vi "activeXtest2015.vi"() -> ()   [LabVIEW 2015]
uses:
  <vilib>/Utility/NIReport.llb/NI_report.lvclass
  <vilib>/addons/_office/NI_ReportGenerationToolkit.lvlib
  <vilib>/Utility/NIReport.llb/Excel/NI_Excel.lvclass
panel:
  out "cell's name":string
  in  "Select Worksheet":i32
  in  "start (-1, -1) 2":cluster{"row":i32, "column":i32}={"row"=-1, "column"=-1}
  out "Worksheet Name":string
  out "Worksheet Names":string[](array[string])
  out "worksheets count":i32
  in  "end (-1, -1)":cluster{"row":i32, "column":i32}={"row"=-1, "column"=-1}
  in  "start (-1, -1)":cluster{"row":i32, "column":i32}={"row"=15, "column"=13}
  in  "report file path":path=path "D:/Cascade/templates/Groundwater Profiling Log_empty_1.xlsx"
  out "error out":errorcluster
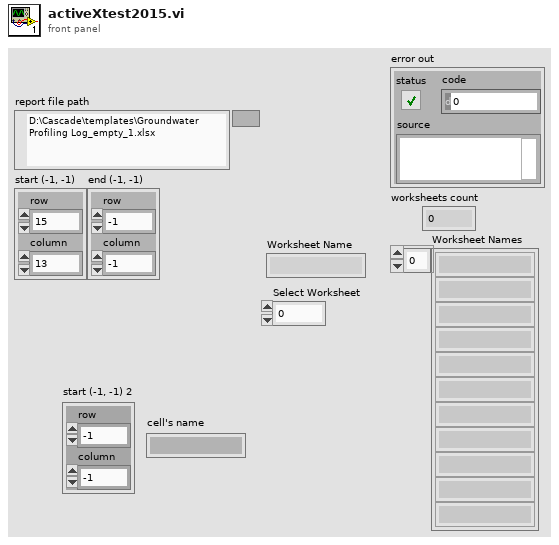
[diagram p1: front panel]
types:
  T1 = enum16{"Standard Report", "HTML", "Word", "Excel"}
  T2 = cluster{"on/off":bool, "weight":i32, "color":u32}
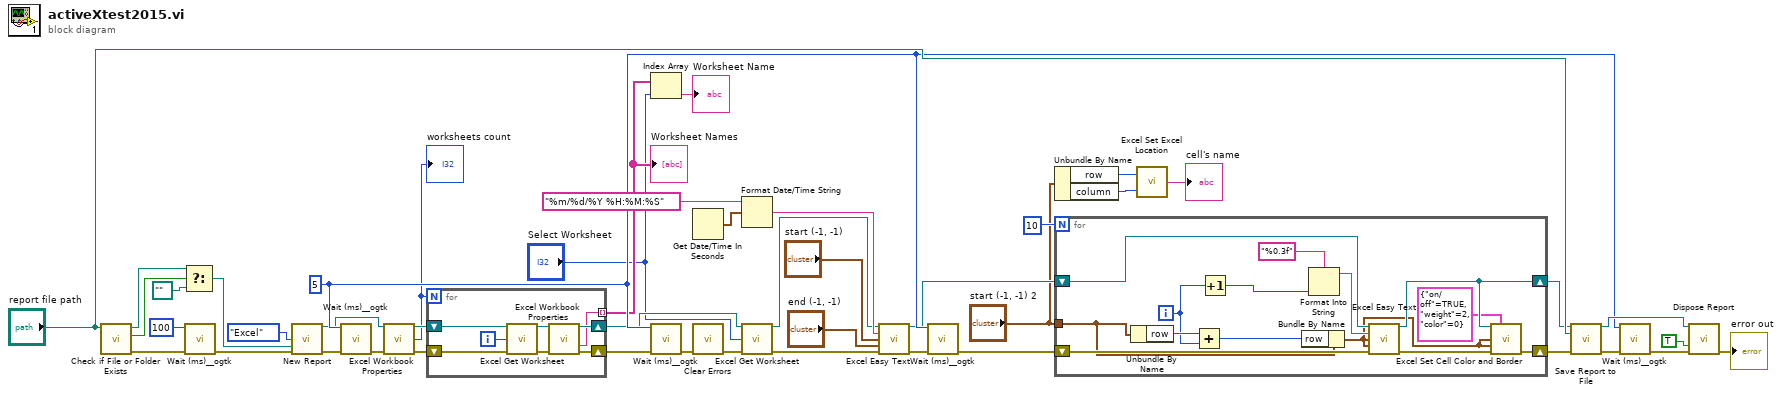
[diagram p0: block diagram]
diagram:
  w24 = u32 5 ("milliseconds to wait")
  n1 = call <vilib>:"Check if File or Folder Exists.vi"("path"="report file path") -> ("error out"=w39:errorcluster, "file or folder exists?"=w38:bool, "dup path"=w37:path)  [unwired: 8 in]
  n2 = Select(t=w37, s=w38, f=path "") -> (s? t:f=w36:path)
  n3 = call <userlib>:"Wait (ms)__ogtk.vi"("error in (no error)"=w39, "milliseconds to wait"=u32 100) -> ("error out"=w23:errorcluster)  [unwired: 8 in, 1 out]
  n4 = call <vilib>:"New Report.vi"("report type"=T1."Excel", "template (empty)"=w36, "error in (no error)"=w23) -> ("report out"=w21:refnum<class "NI_report.lvclass">, "error out"=w33:errorcluster)  [unwired: 11 in]
  n5 = call <userlib>:"Wait (ms)__ogtk.vi"("error in (no error)"=w33, "milliseconds to wait"=w24) -> ("error out"=w20:errorcluster)  [unwired: 8 in, 1 out]
  n6 = call <vilib>:"Excel Workbook Properties.vi"("report in"=w21, "error in (no error)"=w20) -> ("report out"=w18:refnum<class "NI_report.lvclass">, "worksheets count"=w17:i32, "error out"=w19:errorcluster)  [unwired: 10 in, 1 out]
  "worksheets count" <- w17
  n7 = for {
    N: w17 -> [_]
    shift-right: [w47] -> w32
    shift-left: w19 -> [w53]
    shift-right: [w48] -> w14
    shift-left: w18 -> [w52]
    tunnel: [w46] -> w6 mode=indexing
    i -> [w51]
    n8 = call <vilib>:"Excel Get Worksheet.vi"("report in"=w52, "worksheet index (0)"=w51, "error in (no error)"=w53) -> ("report out"=w49:refnum<class "NI_report.lvclass">, "error out"=w50:errorcluster)  [unwired: 11 in]
    n9 = call <vilib>:"Excel Workbook Properties.vi"("report in"=w49, "error in (no error)"=w50) -> ("report out"=w48:refnum<class "NI_report.lvclass">, "current worksheet name"=w46:string, "error out"=w47:errorcluster)  [unwired: 10 in, 1 out]
  }
  "Worksheet Names" <- w6
  n10 = Index Array(array=w6, index="Select Worksheet") -> (element=→"Worksheet Name":string)
  n11 = call <userlib>:"Wait (ms)__ogtk.vi"("error in (no error)"=w32, "milliseconds to wait"=w24) -> ("error out"=w26:errorcluster)  [unwired: 8 in, 1 out]
  n12 = Get Date/Time In Seconds() -> (seconds since 1Jan1904=w31:timestamp)
  n13 = call <vilib>:"Clear Errors.vi"("error in (no error)"=w26) -> ("error out"=w16:errorcluster)  [unwired: 5 in, 1 out]
  n14 = Format Date/Time String(time format string (%c)="%m/%d/%Y %H:%M:%S", seconds (now)=w31) -> (date/time string=w29:string)  [unwired: 1 in]
  n15 = call <vilib>:"Excel Get Worksheet.vi"("report in"=w14, "worksheet index (0)"="Select Worksheet", "error in (no error)"=w16) -> ("report out"=w13:refnum<class "NI_report.lvclass">, "error out"=w15:errorcluster)  [unwired: 11 in]
  n16 = call <vilib>:"Excel Easy Text.vi"("report in"=w13, "text"=w29, "start (-1, -1)"="start (-1, -1)", "end (-1, -1)"="end (-1, -1)", "error in (no error)"=w15) -> ("report out"=w10:refnum<class "NI_report.lvclass">, "error out"=w34:errorcluster)  [unwired: 6 in, 3 out]
  n17 = call <userlib>:"Wait (ms)__ogtk.vi"("error in (no error)"=w34, "milliseconds to wait"=w24) -> ("error out"=w12:errorcluster)  [unwired: 8 in, 1 out]
  n18 = Unbundle By Name("start (-1, -1) 2") -> ("row"=w3:i32, "column"=w2:i32)
  n19 = for {
    N: 10 -> [_]
    shift-right: [w57] -> w11
    shift-left: w12 -> [w67]
    shift-right: [w56] -> w9
    shift-left: w10 -> [w66]
    tunnel: "start (-1, -1) 2" -> [w65]
    i -> [w63]
    n20 = Unbundle By Name(w65) -> ("row"=w64:i32)
    n21 = Add(x=w64, y=w63) -> (x+y=w60:i32)
    n22 = Increment(x=w63) -> (x+1=w59:i32)
    n23 = Bundle By Name(cluster=w65, "row"=w60) -> (w55:cluster{"row":i32, "column":i32})
    n24 = Format Into String(format string="%0.3f", w59) -> (resulting string=w61:string)  [unwired: 2 in, 1 out]
    n25 = call <vilib>:"Excel Easy Text.vi"("report in"=w66, "text"=w61, "start (-1, -1)"=w55, "end (-1, -1)"=w55, "error in (no error)"=w67) -> ("report out"=w56:refnum<class "NI_report.lvclass">, "error out"=w58:errorcluster)  [unwired: 6 in, 3 out]
    n26 = call <vilib>:"Excel Set Cell Color and Border.vi"("report in"=w56, "inside border"=T2 {"on/off"=TRUE, "weight"=2, "color"=0}, "start (-1, -1)"=w55, "end (-1, -1)"=w55, "error in (no error)"=w58) -> ("error out"=w57:errorcluster)  [unwired: 9 in, 1 out]
  }
  n27 = call <vilib>:"Excel Set Excel Location.vi"("column"=w2, "row"=w3) -> ("cell's name"=→"cell's name":string)
  n28 = call-dynamic "Save Report to File.vi"("report in"=w9, "report file path"="report file path", "error in (no error)"=w11) -> ("report out"=w44:refnum<class "NI_report.lvclass">, "error out"=w43:errorcluster)  [unwired: 11 in]
  n29 = call <userlib>:"Wait (ms)__ogtk.vi"("error in (no error)"=w43, "milliseconds to wait"=w24) -> ("error out"=w25:errorcluster)  [unwired: 8 in, 1 out]
  n30 = call-dynamic "Dispose Report.vi"("report in"=w44, "save changes? (F)"=TRUE, "error in (no error)"=w25) -> ("error out"=→"error out":errorcluster)  [unwired: 12 in]
